vi "MK_Write Buffer.vi"(10 "Buffer":string="\u0001", 11 "Handle in":u32) -> (3 "Handle out":u32)   [LabVIEW 2014]
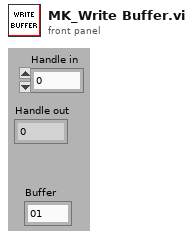
[diagram p1: front panel]
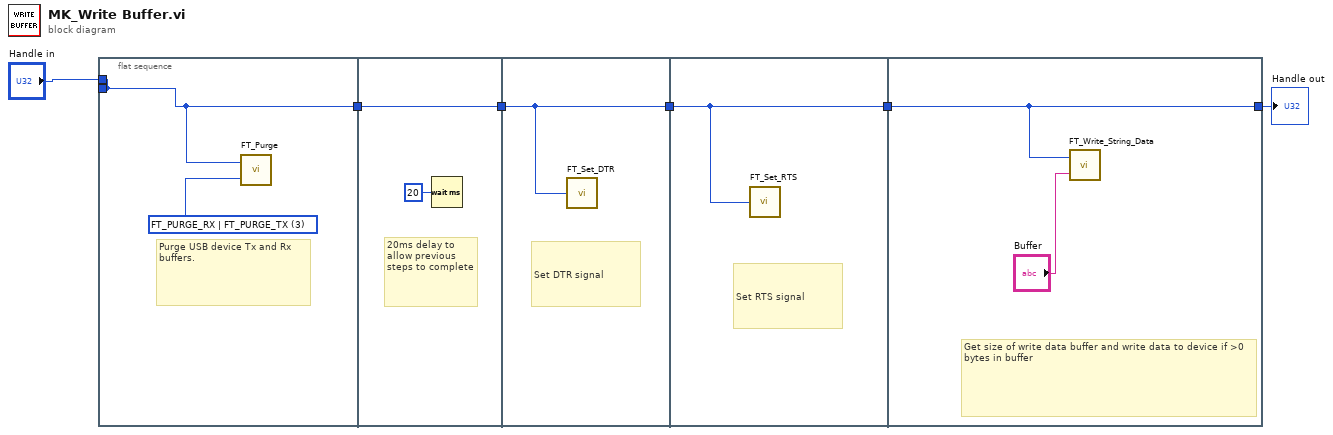
[diagram p0: block diagram]
diagram:
  n1 = flat-sequence {
    tunnel: [w7] -> w6
    tunnel: [w7] -> _
    tunnel: "Handle in" -> [w7]
    tunnel: [w9] -> w5
    tunnel: w6 -> [w9]
    tunnel: w5 -> [w11]
    tunnel: [w11] -> w4
    tunnel: w4 -> [w12]
    tunnel: [w12] -> w3
    tunnel: w3 -> [w13]
    tunnel: [w13] -> w1
    frame #0 {
      w8 = u32 3 items=["FT_PURGE_RX"=1, "FT_PURGE_TX"=2, "FT_PURGE_RX | FT_PURGE_TX"=3] ("Purge Flags")
      # "Purge USB device Tx and Rx buffers."
      n2 = call "FT_Purge.vi"("Purge Flags"=w8, "Handle"=w7) -> ()  [unwired: 1 out]
    }
    frame #1 {
      # "20ms delay to allow previous steps to complete"
      n3 = Wait (ms)(milliseconds to wait=u32 20) -> ()  [unwired: 1 out]
    }
    frame #2 {
      # "Set DTR signal"
      n4 = call "FT_Set_DTR.vi"("Handle"=w11) -> ()  [unwired: 1 out]
    }
    frame #3 {
      # "Set RTS signal"
      n5 = call "FT_Set_RTS.vi"("Handle"=w12) -> ()  [unwired: 1 out]
    }
    frame #4 {
      # "Get size of write data buffer and write data to device if >0 bytes in buffer"
      n6 = call "FT_Write_String_Data.vi"("Buffer"="Buffer", "Handle"=w13) -> ()  [unwired: 2 out]
    }
  }
  "Handle out" <- w1
